vi "getStandardError.vi"(11 "一维数组":dbl[](array[numeric])) -> (3 "标准差":dbl)   [LabVIEW 2017]
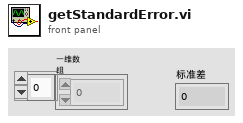
[diagram p1: front panel]
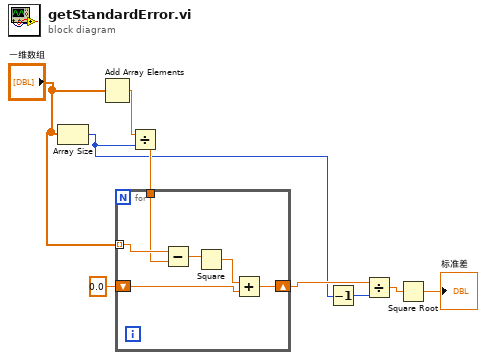
[diagram p0: block diagram]
diagram:
  n1 = Array Size(array="一维数组") -> (size(s)=w3:i32)
  n2 = Add Array Elements(numeric array="一维数组") -> (sum=w9:dbl)
  n3 = Divide(x=w9, y=w3) -> (x/y=w7:dbl)
  n4 = for {
    tunnel: "一维数组" -> [w15] mode=indexing
    tunnel: w7 -> [w14]
    shift-right: [w11] -> w5
    shift-left: 0.0 -> [w10]
    n5 = Subtract(x=w15, y=w14) -> (x-y=w13:dbl)
    n6 = Square(x=w13) -> (x^2=w12:dbl)
    n7 = Add(x=w12, y=w10) -> (x+y=w11:dbl)
  }
  n8 = Decrement(x=w3) -> (x-1=w4:i32)
  n9 = Divide(x=w5, y=w4) -> (x/y=w2:dbl)
  n10 = Square Root(x=w2) -> (sqrt(x)=→"标准差":dbl)
